vi "Handle Command.vi"(8 "error in (no error)":errorcluster, 10 "CMD in":refnum<class "Update Blue DC.lvclass">, 11 "Object In":refnum<class>) -> (0 "error out":errorcluster, 1 "Command Successful?":bool, 2 "CMD out":refnum<class "Update Blue DC.lvclass">, 3 "Object Out":refnum<class>)   [LabVIEW 2014, in "eCRDS Library.lvlib" / "Update Blue DC.lvclass"]
doc: "This VI will contain the code used to actually execute the request. If the request is successful, this will be indicated by the boolean output <b>Command Successful?</b>. The boolean output can then be used by the <b>Command Reply</b> which sends a reply if the reply queue is valid."
uses:
  Update Blue DC.lvclass
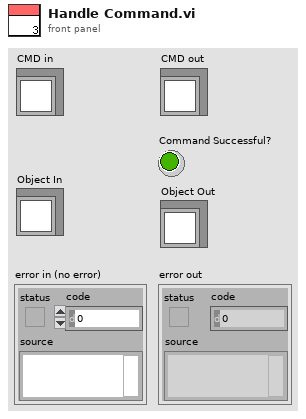
[diagram p1: front panel]
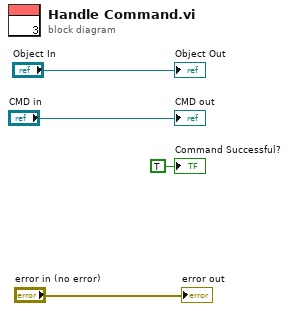
[diagram p0: block diagram]
diagram:
  "error out" <- "error in (no error)"
  "CMD out" <- "CMD in"
  "Object Out" <- "Object In"
  "Command Successful?" <- TRUE ("Command Successful?")
